vi "write_text_file.vi"(1 "name":string, 2 "base path":path) -> ()   [LabVIEW 2013]
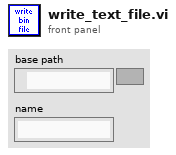
[diagram p1: front panel]
types:
  T1 = enum16{"open", "replace", "create", "open or create", "replace or create", "replace or create with confirmation"}
  T2 = cluster{"Xpixels":i32, "Vx-min ref":dbl, "Vx-max ref":dbl, "P":dbl, "Ypixels":i32, "Vy-min ref":dbl, "Vy-max ref":dbl, "srate":sgl, "sAOxy":i32, "timeout":dbl, "type":string, "date":string, "time":string, "Colormap":u16, "Drawing Mode":u16, "Scanning Mode":u16, "square pixels":bool, "square matrix":bool, "Xpixels Img":i32, "Vx-min Img":dbl, "VX-max Img":dbl, "Ypixels Img":i32, "Vy-min Img":dbl, "Vy-max Img ":dbl, "Angle Img":dbl, "autoshutter":bool, "finite":bool, "cont":bool, "wavdet":bool, "measpoints":i32, "avpp":i32, "bufferAO":i32, "bufferAI":i32, "CH1":bool, "CH2":bool, "X":bool, "Y":bool, "Ip":bool, "Vp":bool, "starttick":u32, "waveform":path, "Vx-ref":dbl, "Vy-ref":dbl, "refreshrate":dbl, "refreshbuffer":i32, "tt_cycles":i32, "motorref":refnum<k7>, "mirrorswitch":refnum<k7>, "sample mode":i32, "maxbufferAI":i32, "sampletreshold":dbl}
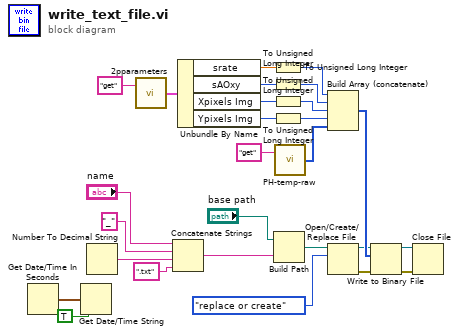
[diagram p0: block diagram]
diagram:
  n1 = Get Date/Time In Seconds() -> (seconds since 1Jan1904=w2:timestamp)
  n2 = Get Date/Time String(seconds (now)=w2, want seconds? (F)=TRUE) -> ()  [unwired: 1 in, 2 out]
  n3 = Number To Decimal String() -> (number=w25:i32, decimal integer string=w21:string)  [unwired: 1 in]
  n4 = call "2pparameters.vi"("command"="get") -> ("Params out"=w18:T2)  [unwired: 1 in]
  n5 = Concatenate Strings("name", "_" ("command"), w21, ".txt" ("string")) -> (w26:string)
  n6 = Unbundle By Name(w18) -> ("srate"=w15:sgl, "sAOxy"=w14:i32, "Xpixels Img"=w12:i32, "Ypixels Img"=w10:i32)
  n7 = To Unsigned Long Integer(number=w15) -> (unsigned 32bit integer=w17:u32)
  n8 = To Unsigned Long Integer(number=w14) -> (unsigned 32bit integer=w13:u32)
  n9 = To Unsigned Long Integer(number=w12) -> (unsigned 32bit integer=w11:u32)
  n10 = To Unsigned Long Integer(number=w10) -> (unsigned 32bit integer=w9:u32)
  n11 = Build Path(base path="base path", name or relative path=w26) -> (appended path=w24:path)
  n12 = call "PH-temp-raw.vi"("command"="get") -> ("array out"=w8:u32[])  [unwired: 1 in]
  n13 = Build Array (concatenate)(w17, w13, w11, w9, w8) -> (w7:u32[])
  n14 = Open/Create/Replace File(file path (use dialog)=w24, operation (0:open)=T1."replace or create") -> (refnum out=w6:refnum<file>, error out=w5:errorcluster)  [unwired: 4 in, 1 out]
  n15 = Write to Binary File(file (use dialog)=w6, data=w7, error in=w5) -> (refnum out=w3:refnum<file>, error out=w4:errorcluster)  [unwired: 3 in, 1 out]
  n16 = Close File(refnum=w3, error in=w4) -> ()  [unwired: 2 out]
